vi "BuildMenu.vi"(8 "error in (no error)":errorcluster, 10 "menu reference":refnum<k9>, 11 "AI_Task in":refnum<class "AI_Task.lvclass">) -> (0 "error out":errorcluster, 3 "AI_Task out":refnum<class "AI_Task.lvclass">)   [LabVIEW 2025, in "AI_Task.lvlib" / "AI_Task.lvclass"]
uses:
  AI_Task.lvclass
  AI_Task.lvclass/AI_Task.ctl
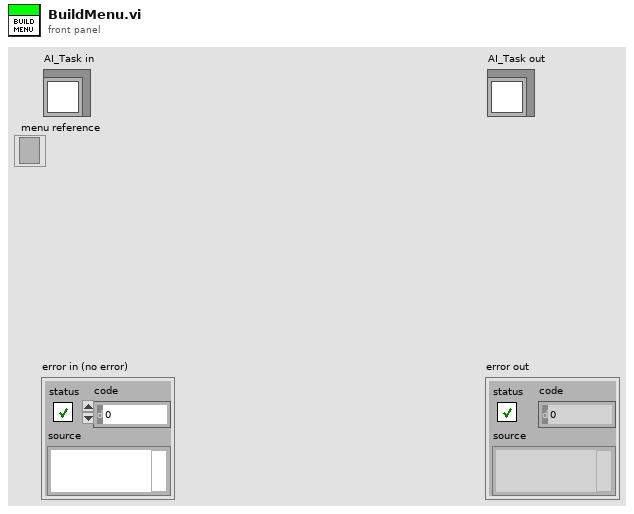
[diagram p1: front panel]
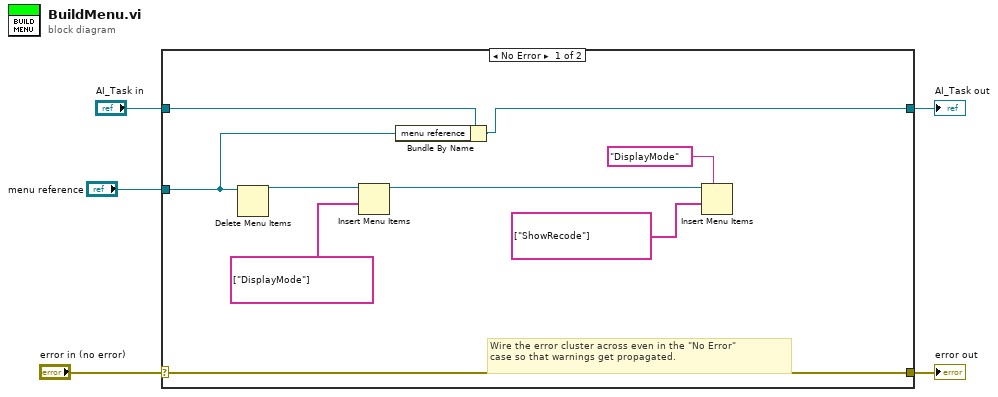
[diagram p0: block diagram]
diagram:
  n1 = case shown="No Error" "error in (no error)" {
    selector: "error in (no error)" -> [w14 w16]
    tunnel: [w14 w16] -> w4
    tunnel: [w10 w15] -> w2
    tunnel: "AI_Task in" -> [w12 w15]
    tunnel: "menu reference" -> [w11 _]
    frame No Error {
      # "Wire the error cluster across even in the \"No Error\"\ncase so that warnings get propagated."
      n2 = Delete Menu Items(9:w11) -> (3:w9:refnum<k9>)  [unwired: 3 in, 1 out]
      n3 = Insert Menu Items(7:string[] ["DisplayMode"] ("item tags"), 9:w9) -> (3:w8:refnum<k9>)  [unwired: 4 in, 2 out]
      n4 = Bundle By Name(cluster=w12, "menu reference"=w11) -> (w10:refnum<class "AI_Task.lvclass">)
      n5 = Insert Menu Items(5:"DisplayMode" ("menu tag"), 7:string[] ["ShowRecode"] ("item tags"), 9:w8) -> ()  [unwired: 3 in, 3 out]
    }
    frame Error {
    }
  }
  "error out" <- w4
  "AI_Task out" <- w2
